vi "TempDAQFGV.vi"(7 "Ctrl":enum16{"Init", "Start", "Read", "Stop", "Exit"}(ring), 8 "error in (no error)":errorcluster caption="에러 입력(에러 없음)") -> (0 "error out":errorcluster caption="에러 출력", 2 "data":dbl[](array[numeric]))   [LabVIEW 2023, in "DAQ Module.lvlib"]
uses:
  DAQ Module.lvlib
  <vilib>/numeric/Random Number (Range) DBL.vi
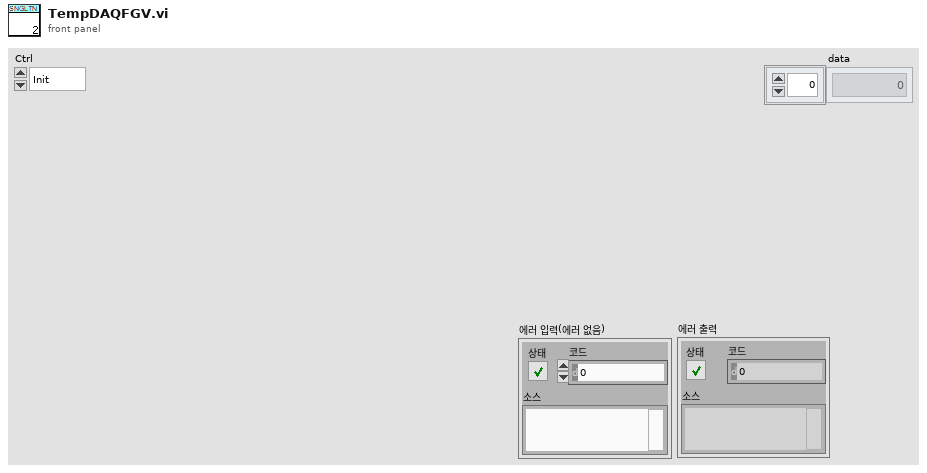
[diagram p1: front panel]
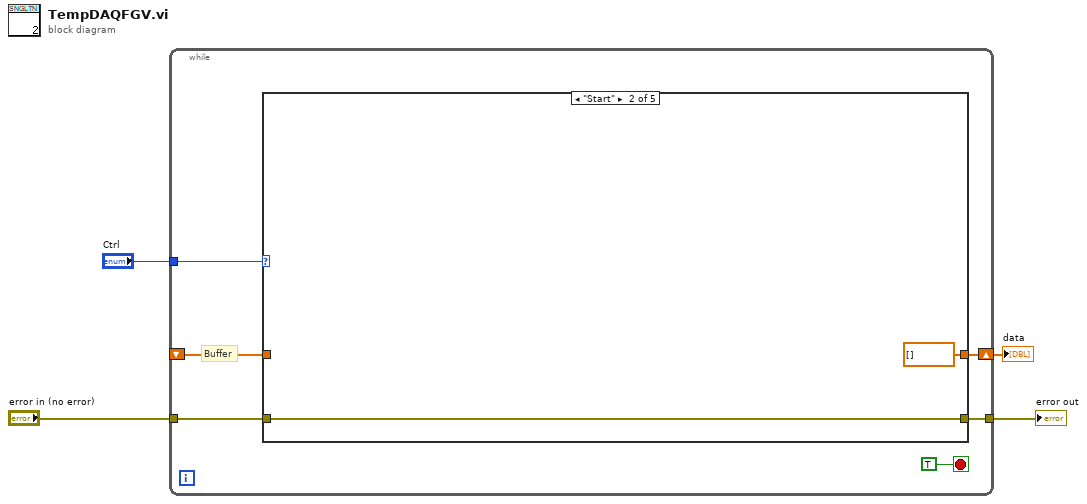
[diagram p0: block diagram]
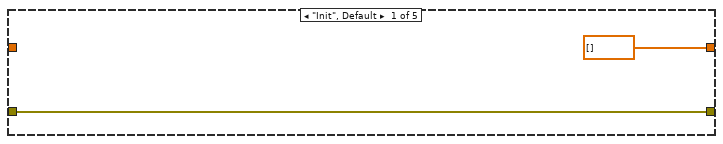
[diagram p2: hidden frame]
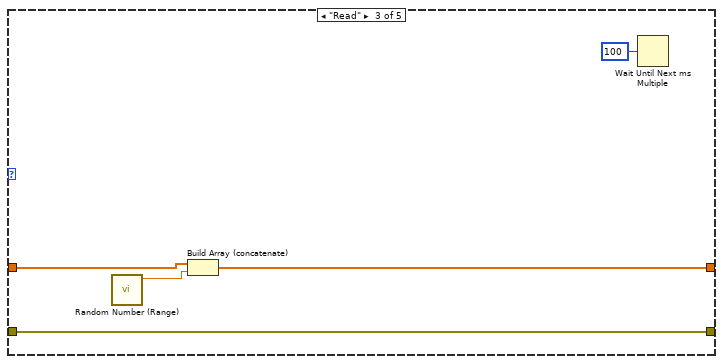
[diagram p3: hidden frame]
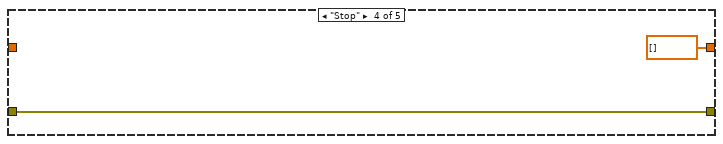
[diagram p4: hidden frame]
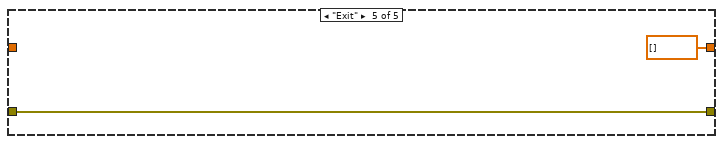
[diagram p5: hidden frame]
diagram:
  n1 = while {
    tunnel: "Ctrl" -> [w10]
    shift-right: [w8] -> w3
    shift-left: _ -> [w7]
    tunnel: "error in (no error)" -> [w6]
    tunnel: [w5] -> w1
    stop <- TRUE stop-if-true
    # "Buffer"
    n2 = case shown="\"Start\"" w10 {
      tunnel: [dbl[] [] dbl[] [] w19 dbl[] [] dbl[] []] -> w8
      tunnel: w7 -> [_ _ w16 _ _]
      tunnel: w6 -> [w11 w13 w17 w20 w22]
      tunnel: [w11 w13 w17 w20 w22] -> w5
      frame "Init", Default {
      }
      frame "Start" {
      }
      frame "Read" {
        n3 = call-poly <vilib>:"Random Number (Range).vi"() -> ("number"=w15:dbl)  [unwired: 11 in]
        n4 = Build Array (concatenate)(w16, w15) -> (w19:dbl[])
        n5 = Wait Until Next ms Multiple(millisecond multiple=u32 100 ("ms 배수")) -> ()  [unwired: 1 out]
      }
      frame "Stop" {
      }
      frame "Exit" {
      }
    }
  }
  "data" <- w3
  "error out" <- w1
